vi "NetComm_getJoystickAxes.vi"(8 "error in (no error)":errorcluster, 11 "Joystick Number":i32) -> (0 "error out":errorcluster, 2 "Axes":i16[](array[numeric]))   [LabVIEW 2017]
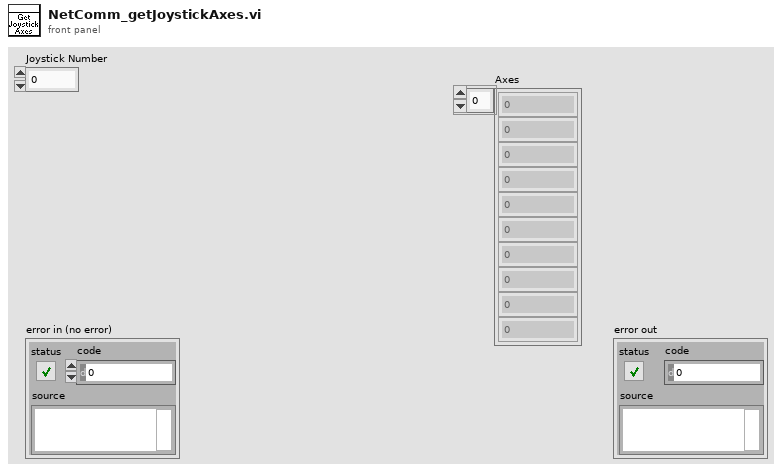
[diagram p1: front panel]
types:
  T1 = enum16{"big-endian, network order", "native, host order", "little-endian"}
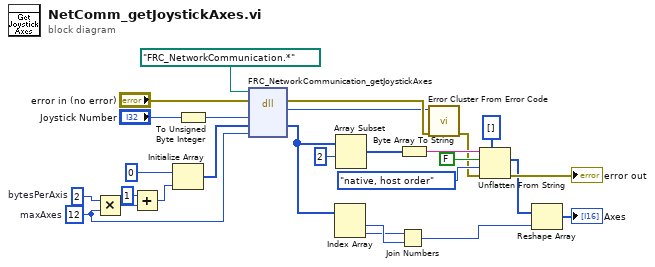
[diagram p0: block diagram]
diagram:
  w20 = u8 2  # bytesPerAxis
  w15 = u8 12  # maxAxes
  n1 = Multiply(x=w20, y=w15) -> (x*y=w19:u8)
  n2 = Add(x=u8 1, y=w19) -> (x+y=w17:u8)
  n3 = Initialize Array(u8 0, w17) -> (w16:u8[])
  n4 = To Unsigned Byte Integer(number="Joystick Number") -> (unsigned 8bit integer=w22:u8)
  n5 = dll-call lib="?" fn="FRC_NetworkCommunication_getJoystickAxes"(path in=path "FRC_NetworkCommunication.*", error in="error in (no error)", "joystickNum"=w22, "axes"=w16, "maxAxes"=w15) -> (error out=w25:errorcluster, "return type"=w24:i32, "axes"=w6:u8[])  [unwired: 3 in, 1 out]
  n6 = Index Array(array=w6) -> (element #1=w3:u8, element #2=w2:u8)  [unwired: 2 in]
  n7 = Array Subset(array=w6, index=2) -> (w8:u8[])  [unwired: 1 in]
  n8 = Join Numbers(hi=w2, lo=w3) -> ((hi.lo)=w1:u16)
  n9 = Byte Array To String(unsigned byte array=w8) -> (string=w13:string)
  n10 = call <vilib>:"Error Cluster From Error Code.vi"("error in (no error)"=w25, "error code (0)"=w24) -> ("error out"=w10:errorcluster)  [unwired: 7 in]
  n11 = Unflatten From String(type=i16[] [], binary string=w13, data includes array or string size? (T)=FALSE, byte order (0:big-endian, network order)=T1."native, host order", error in (no error)=w10) -> (value=w5:i16[], error out=→"error out":errorcluster)  [unwired: 1 out]
  n12 = Reshape Array(w5, w1) -> (→"Axes":i16[])
